vi "Read Power Limits.vi"   [LabVIEW 2023, in "Power Limits.lvclass"]
uses:
  Power Limits.lvclass
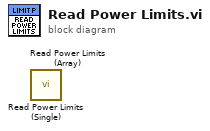
[diagram p0: block diagram]
diagram:
  n1 = call "Read Power Limits (Single).vi"() -> ()  [unwired: 7 in, 5 out]
  n2 = call "Read Power Limits (Array).vi"() -> ()  [unwired: 7 in, 5 out]
